vi "wahooPIP.vi"(8 "error in (no error)":errorcluster) -> (0 "error out":errorcluster, 3 "WAHOO-22":string)   [LabVIEW 2018]
uses:
  Global_1259.vi
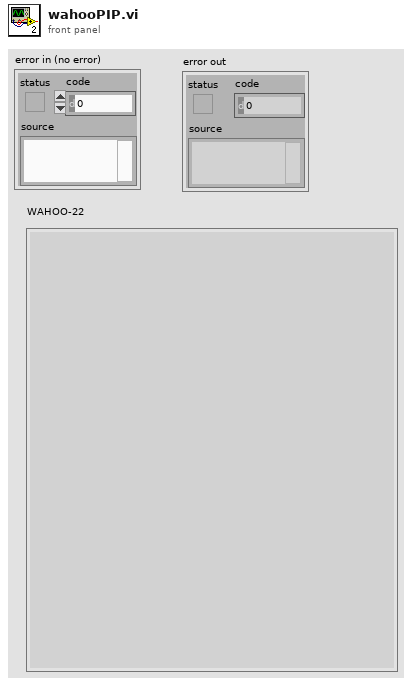
[diagram p1: front panel]
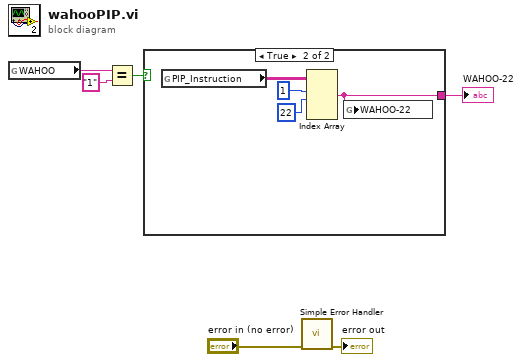
[diagram p0: block diagram]
diagram:
  n1 = global read "Global_1259.vi" "WAHOO"() -> (w6:string)
  n2 = Equal?(x=w6, y="1") -> (x = y?=w4:bool)
  n3 = case shown="True" w4 {
    tunnel: [_ w7] -> w3
    frame False {
    }
    frame True {
      n4 = global read "Global_1259.vi" "PIP_Instruction"() -> (w10:string[][])
      n5 = Index Array(array=w10, index (row) #1=1 ("index (row)"), index (col) #1=22 ("disabled index (col)")) -> (element #1=w7:string)  [unwired: 2 in, 1 out]
      n6 = global write "Global_1259.vi" "WAHOO-22"(w7) -> ()
    }
  }
  "WAHOO-22" <- w3
  n7 = call <vilib>:"Simple Error Handler.vi"("error in (no error)"="error in (no error)") -> ("error out"=→"error out":errorcluster)  [unwired: 4 in, 4 out]
